vi "SaveResultToFile.vi"(11 "Sequence Context In":refnum<k7>) -> (0 "error out":errorcluster, 3 "Report Text":string)   [LabVIEW 2018]
uses:
  <vilib>/Utility/file.llb/Write Delimited Spreadsheet (string).vi
panel:
  out "Array":string[](array[string])
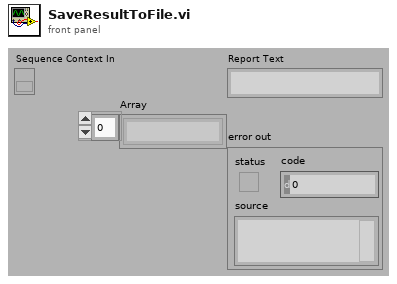
[diagram p1: front panel]
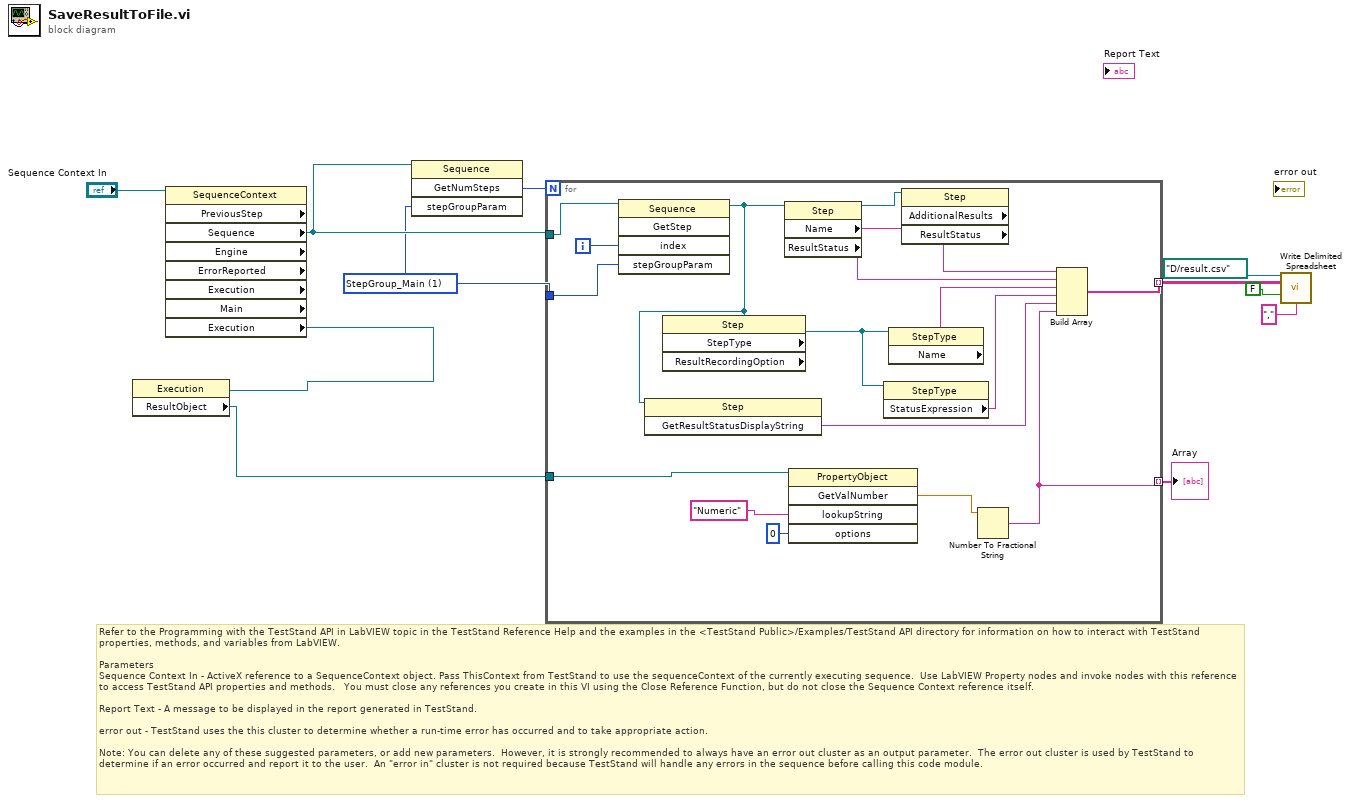
[diagram p0: block diagram]
diagram:
  w8 = 1 items=["StepGroup_Setup", "StepGroup_Main", "StepGroup_Cleanup"] ("stepGroupParam")
  # "Refer to the Programming with the TestStand API in LabVIEW topic in the TestStand Reference Help and the examples in the <TestStand Public>/Examples/TestStand API directory for information on how to interact with TestStand properties, methods, and variables from LabVIEW.\n\nParameters\nSequence Context In - ActiveX reference to a SequenceContext object. Pass ThisContext from TestStand to use the sequenceContext of the currently executing sequence.  Use LabVIEW Property nodes and invoke nodes with this reference to access TestStand API properties and methods.   You must close any references you create in this VI using the Close Reference Function, but do not close the Sequence Context reference itself.\n\nReport Text - A message to be displayed in the report generated in TestStand. \n\nerror out - TestStand uses the this cluster to determine whether a run-time error has occurred and to take appropriate action.  \n\nNote: You can delete any of these suggested parameters, or add new parameters.  However, it is strongly recommended to always have an error out cluster as an output parameter.  The error out cluster is used by TestStand to determine if an error occurred and report it to the user.  An \"error in\" cluster is not required because TestStand will handle any errors in the sequence before calling this code module."
  n1 = property class="SequenceContext" props=["PreviousStep", "Sequence", "Engine", "ErrorReported", "Execution", "Main", "Execution"](reference="Sequence Context In") -> ("Sequence"=w9:refnum<k7>, "Execution"=w3:refnum<k7>)  [unwired: 1 in, 7 out]
  n2 = property class="Execution"(reference=w3) -> ("ResultObject"=w2:refnum<k7>)  [unwired: 1 in, 2 out]
  n3 = invoke class="Sequence" method="GetNumSteps"(reference=w9, "stepGroupParam"=w8) -> ("GetNumSteps"=w7:i32)  [unwired: 2 in, 3 out]
  n4 = for {
    N: w7 -> [_]
    tunnel: [w28] -> w6 mode=indexing
    tunnel: w9 -> [w25]
    tunnel: w8 -> [w24]
    tunnel: w2 -> [w16]
    tunnel: [w14] -> w1 mode=indexing
    i -> [w23]
    n5 = invoke class="Sequence" method="GetStep"(reference=w25, "index"=w23, "stepGroupParam"=w24) -> ("GetStep"=w21:refnum<k7>)  [unwired: 2 in, 4 out]
    n6 = invoke class="Step" method="GetResultStatusDisplayString"(reference=w21) -> ("GetResultStatusDisplayString"=w18:string)  [unwired: 2 in, 2 out]
    n7 = property class="Step" props=["StepType", "ResultRecordingOption"](reference=w21) -> ("StepType"=w19:refnum<k7>)  [unwired: 1 in, 3 out]
    n8 = property class="Step"(reference=w21) -> (reference out=w17:refnum<k7>, "Name"=w27:string, "ResultStatus"=w26:string)  [unwired: 1 in, 1 out]
    n9 = invoke class="PropertyObject" method="GetValNumber"(reference=w16, "lookupString"="Numeric", "options"=0) -> ("GetValNumber"=w15:dbl)  [unwired: 2 in, 4 out]
    n10 = property class="StepType"(reference=w19) -> ("StatusExpression"=w20:string)  [unwired: 1 in, 2 out]
    n11 = property class="StepType"(reference=w19) -> ("Name"=w22:string)  [unwired: 1 in, 2 out]
    n12 = property class="Step" props=["AdditionalResults", "ResultStatus"](reference=w17) -> ()  [unwired: 1 in, 4 out]
    n13 = Number To Fractional String(number=w15) -> (F-format string=w14:string)  [unwired: 3 in]
    n14 = Build Array(w27, w26, w22, w20, w18, w14) -> (w28:string[])
  }
  "Array" <- w1
  n15 = call-poly <vilib>:"Write Delimited Spreadsheet.vi"("file path (dialog if empty)"=path "D:/result.csv", "2D data"=w6, "append to file? (new file:F)"=FALSE, "delimiter (\\t)"="," ("delimiter (\\t)")) -> ()  [unwired: 10 in, 2 out]
